vi "CL3IF_GetTrendData.vi"(8 "error in":errorcluster {"code" format="%x"}, 9 "requestDataCount":u32, 10 "index":u32, 11 "deviceId":i32) -> (0 "error out":errorcluster {"code" format="%x"}, 1 "obtainedDataCount":u32, 2 "nextIndex":u32, 3 "measurementData":T1[](array[typedef]) {"outMeasurementData"."judgeResult" items=["HI"=1, "GO"=2, "LO"=4]}, 5 "outTarget":T5 items=["OUT01"=1, "OUT02"=2, "OUT03"=4, "OUT04"=8, "OUT05"=16, "OUT06"=32, "OUT07"=64, "OUT08"=128, "ALL OUT"=255])   [LabVIEW 2020, in "Keyence CL-3000.lvlib"]
doc: "This function is used to get all the measurement values buffered on the device. The calculation shown below is used to find the upper limit of the amount of data that can be obtained. If a request is made for an amount of data that exceeds this upper limit, an amount of data equivalent to the upper limit is returned.\nCalculation: 307,130  (32 + 8 ~ measurement target OUT count)"
uses:
  Keyence CL-3000.lvlib
  enums/CL3IF_OUTNO.ctl
  clusters/CL3IF_MEASUREMENT_DATA.ctl
  clusters/CL3IF_OUTMEASUREMENT_DATA.ctl
  enums/CL3IF_VALUE_INFO.ctl
  enums/CL3IF_JUDGE_RESULT.ctl
  Private/enums/Function Name.ctl
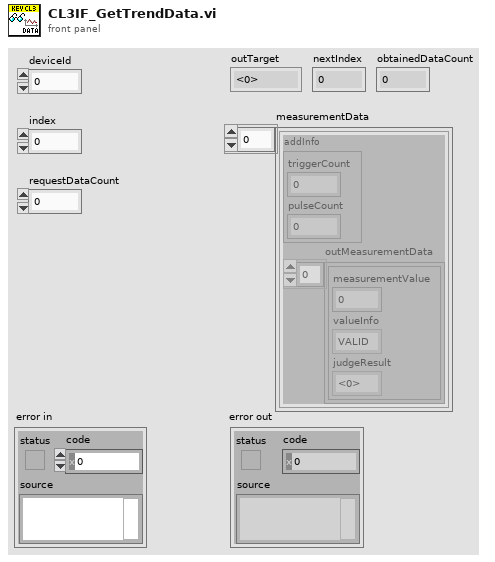
[diagram p1: front panel]
types:
  T1 = typedef "Keyence CL-3000.lvlib/CL3IF_MEASUREMENT_DATA.ctl" = cluster{"addInfo":cluster{"triggerCount":u32, "pulseCount":i32}, "outMeasurementData":T2[]}
  T2 = typedef "Keyence CL-3000.lvlib/CL3IF_OUTMEASUREMENT_DATA.ctl" = cluster{"measurementValue":i32, "valueInfo":T3, "judgeResult":T4}
  T3 = typedef "Keyence CL-3000.lvlib/CL3IF_VALUE_INFO.ctl" = enum8{"VALID", "JUDGMENTSTANDBY", "INVALID", "OVERDISPRANGE_P", "OVERDISPRANGE_N"}
  T4 = typedef "Keyence CL-3000.lvlib/CL3IF_JUDGE_RESULT.ctl" = u8
  T5 = typedef "Keyence CL-3000.lvlib/CL3IF_OUTNO.ctl" = u16
  T6 = typedef "Keyence CL-3000.lvlib/Function Name.ctl" = enum16{"Initialize", "Close", "CL3IF_GetMeasurementData", "CL3IF_GetTrendIndex", "CL3IF_GetTrendData", "CL3IF_GetStorageIndex", "CL3IF_GetStorageData", "CL3IF_AutoZeroMulti", "CL3IF_AutoZeroGroup", "CL3IF_TimingMulti", "CL3IF_TimingGroup", "CL3IF_ResetMulti", "CL3IF_ResetGroup", "CL3IF_LightControl", "CL3IF_MeasurementControl", "CL3IF_SwitchProgram", "CL3IF_GetProgramNo", "CL3IF_StartStorage", "CL3IF_StopStorage", "CL3IF_ClearStorageData", "CL3IF_GetPulseCount", "CL3IF_ResetPulseCount", "CL3IF_GetLightWaveform"}
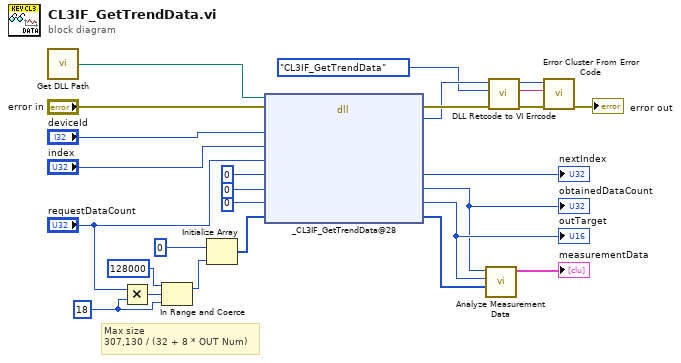
[diagram p0: block diagram]
diagram:
  w4 = u32 18 ("data size")
  # "Max size\n307,130 / (32 + 8 * OUT Num)"
  n1 = call "Get DLL Path.vi"() -> ("DLL Path"=w22:path)  [unwired: 1 in]
  n2 = Multiply(x="requestDataCount", y=w4) -> (x*y=w6:u32)
  n3 = In Range and Coerce(upper limit=u32 128000 ("size"), x=w6, lower limit=w4) -> (coerced(x)=w3:u32)  [unwired: 1 out]
  n4 = Initialize Array(u32 0, w3) -> (w8:u32[])
  n5 = dll-call lib="C:/Program Files (x86)/National Instruments/LabVIEW 2018/instr.lib/Keyence CL-3000/CL3_IF.dll" fn="_CL3IF_GetTrendData@28"(path in=w22, error in="error in", "deviceid"="deviceId", "index"="index", "requestDataCount"="requestDataCount", "nextIndex"=u32 0, "obtainedDataCount"=u32 0, "outTarget"=u16 0, "measurementData"=w8) -> (error out=w19:errorcluster, "RC"=w18:i32, "nextIndex"=→"nextIndex":u32, "obtainedDataCount"=w15:u32, "outTarget"=w16:u16, "measurementData"=w7:u32[])  [unwired: 4 in, 1 out]
  "obtainedDataCount" <- w15
  "outTarget" <- w16
  n6 = call "Analyze Measurement Data.vi"("measurementData"=w7, "outTarget"=w16, "obtainedDataCount"=w15) -> ("MEASUREMENT_DATA"=→"measurementData":T1[])  [unwired: 8 in]
  n7 = call "DLL Retcode to VI Errcode.vi"("error in (no error)"=w19, "Function Name"=Function_Name."CL3IF_GetTrendData", "DLL Retcode"=w18) -> ("error out"=w26:errorcluster, "ErrorMessage"=w1:string, "VI Errcode"=w25:i32)  [unwired: 6 in]
  n8 = call <vilib>:"Error Cluster From Error Code.vi"("error in (no error)"=w26, "error message (\"\")"=w1, "error code (0)"=w25) -> ("error out"=→"error out":errorcluster)  [unwired: 6 in]
